vi "Log State JKI.vi"(0 "Current State In":string, 5 "Arguments In":string, 7 "Error In (no error)":errorcluster, 9 "StatesToIgnore":string[](array[string]), 11 "StatesForTraceLevel":string[](array[string]), 13 "EnableLogging?":bool) -> (6 "Current State":string, 8 "Arguments":string)   [LabVIEW 2020, in "TaskfileRunner Tool.lvlib"]
doc: "Log the state and arguments of the current state and also the error of the previous state of the JKI State Machine 2024 usually using the DEBUG log level.\nStates that are listed in the StatesForTraceLevel Input are logged with a log level of TRACE.\nStates that are listed in the StatesToIgnore are not logged.\n\nIt is important to use the JKI State Machine 2024"
uses:
  <vilib>/Utility/error.llb/DialogType.ctl
  16354a92-b9ac-49f3-ab46-e17f0121f75c.vi
  3b7a71ad-25d6-447f-a954-168ecec1f7c2.vi
  16354a92-b9ac-49f3-ab46-e17f0121f75c.vi/ff40df25-0e41-4205-825d-56c19dc320b6.vi
  3b7a71ad-25d6-447f-a954-168ecec1f7c2.vi/ff40df25-0e41-4205-825d-56c19dc320b6.vi
  <vilib>/Utility/Debug Log/Display.vi
  <vilib>/regexp/Match Regular Expression.xnode
  TaskfileRunner Tool.lvlib
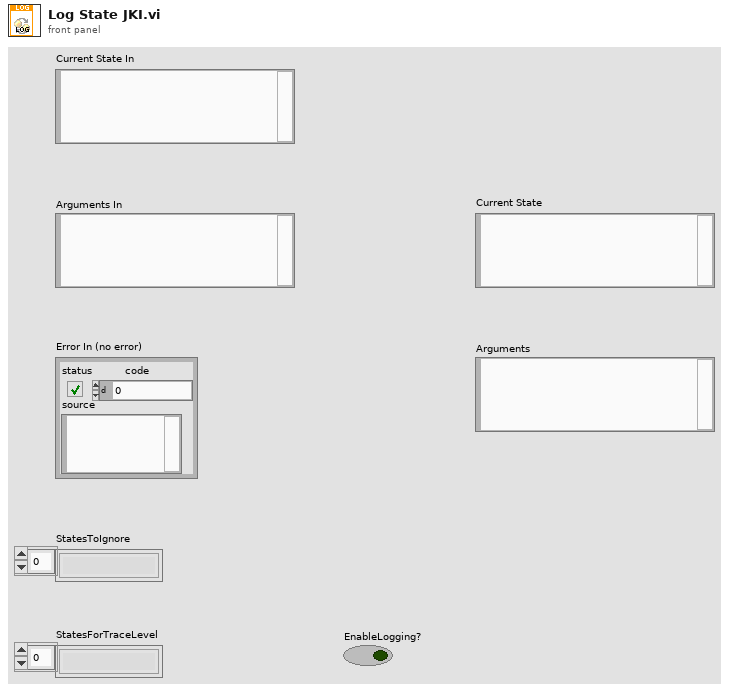
[diagram p1: front panel]
types:
  T1 = typedef "DialogType.ctl" = u16
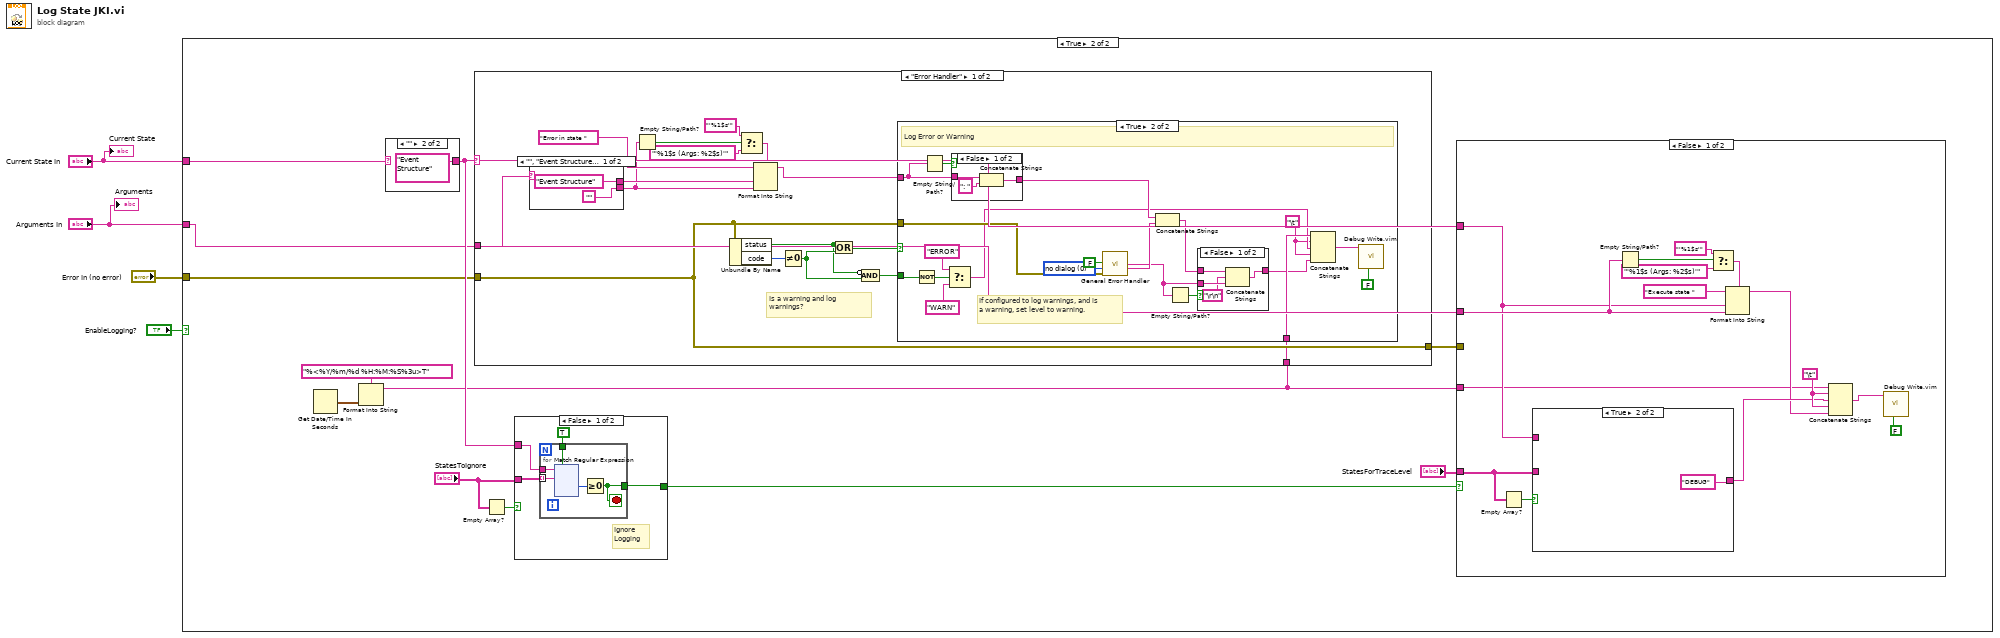
[diagram p0: block diagram]
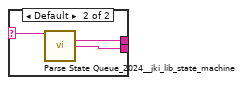
[diagram p6: hidden frame]
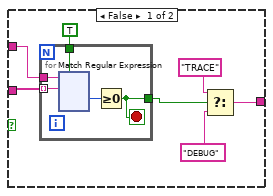
[diagram p10: hidden frame]
diagram:
  n1 = case shown="True" "EnableLogging?" {
    tunnel: "Current State In" -> [_ w12]
    tunnel: "Arguments In" -> [_ w11]
    tunnel: "Error In (no error)" -> [_ w10]
    frame False {
    }
    frame True {
      n2 = Get Date/Time In Seconds() -> (seconds since 1Jan1904=w7:timestamp)
      n3 = Format Into String(format string="%<%Y/%m/%d %H:%M:%S%3u>T", w7) -> (resulting string=w5:string)  [unwired: 2 in, 1 out]
      n4 = case shown="\"\"" w12 {
        selector: w12 -> [w68 _]
        tunnel: [w68 "Event Structure"] -> w14
        frame Default {
        }
        frame "" {
        }
      }
      n5 = case shown="\"Error Handler\"" w14 {
        tunnel: w11 -> [w30 _]
        tunnel: w10 -> [w18 w67]
        tunnel: [w18 w67] -> w8
        tunnel: w5 -> [w17 _]
        frame "Error Handler" {
          # "Is a warning and log warnings?"
          n6 = case shown="\"\", \"Event Structure\"" w30 {
            selector: w30 -> [_ w64]
            tunnel: ["Event Structure" ("Current State") w66] -> w32
            tunnel: ["" w65] -> w29
            frame "", "Event Structure" {
            }
            frame Default {
              n7 = call <vilib>:"Parse State Queue_2024__jki_lib_state_machine.vi"("State Queue"=w64) -> ("Current State"=w66:string, "Arguments"=w65:string)  [unwired: 12 in, 1 out]
            }
          }
          n8 = Empty String/Path?(string/path=w29) -> (empty?=w28:bool)
          n9 = Unbundle By Name(w18) -> ("status"=w22:bool, "code"=w24:i32)
          n10 = Select(t="'%1$s'" ("format string"), s=w28, f="'%1$s (Args: %2$s)'" ("format string")) -> (s? t:f=w25:string)
          n11 = Format Into String(format string=w25, initial string="Error in state ", w32, w29) -> (resulting string=w19:string)  [unwired: 1 in, 1 out]
          n12 = Not Equal To 0?(x=w24) -> (x != 0?=w23:bool)
          n13 = Or(x=w22, y=w23) -> (x .or. y?=w20:bool)
          n14 = Compound Arithmetic op=AND(invert w22, w23) -> (w21:bool)
          n15 = case shown="True" w20 {
            tunnel: w18 -> [_ w47]
            tunnel: w21 -> [_ w52]
            tunnel: w19 -> [_ w50]
            tunnel: w17 -> [_ w38]
            frame False {
              # "No error/not configured to log warnings, do nothing."
            }
            frame True {
              w36 = "\t"
              w46 = T1 0 items=["no dialog", "OK message", "continue or stop message", "OK message + warnings", "continue/stop + warnings"] ("type of dialog (OK msg:1)")
              # "If configured to log warnings, and is a warning, set level to warning."
              # "Log Error or Warning"
              n16 = Not(x=w52) -> (.not. x?=w51:bool)
              n17 = Empty String/Path?(string/path=w50) -> (empty?=w48:bool)
              n18 = Select(t="ERROR", s=w51, f="WARN") -> (s? t:f=w37:string)
              n19 = case shown="False" w48 {
                tunnel: w50 -> [w60 w61]
                tunnel: [w58 w61] -> w49
                frame False {
                  n20 = Concatenate Strings(w60, ": " ("string")) -> (w58:string)
                }
                frame True {
                }
              }
              n21 = call <vilib>:"General Error Handler.vi"("search ni.com link visible?(T)"=FALSE, "type of dialog (OK msg:1)"=w46, "error in (no error)"=w47) -> ("source out"=w42:string, "message"=w44:string)  [unwired: 8 in, 3 out]
              n22 = Concatenate Strings(w49, w44) -> (w34:string)
              n23 = Empty String/Path?(string/path=w42) -> (empty?=w43:bool)
              n24 = case shown="False" w43 {
                tunnel: w42 -> [w54 _]
                tunnel: [w56 w57] -> w35
                tunnel: w34 -> [w55 w57]
                frame False {
                  n25 = Concatenate Strings(w55, "\r\n", w54) -> (w56:string)
                }
                frame True {
                }
              }
              n26 = Concatenate Strings(w38, w36, w37, w36, w35) -> (w33:string)
              n27 = call "Debug Write.vim"("include timestamp? (F)"=FALSE, "value"=w33) -> ()  [unwired: 9 in, 1 out]
            }
          }
        }
        frame Default {
        }
      }
      n28 = Empty Array?(array="StatesToIgnore") -> (empty?=w16:bool)
      n29 = case shown="False" w16 {
        tunnel: "StatesToIgnore" -> [w73 _]
        tunnel: w14 -> [w72 _]
        tunnel: [w70 _] -> w13
        frame False {
          # "Ignore\nLogging"
          n30 = for {
            tunnel: [w77] -> w70
            tunnel: w73 -> [w76] mode=indexing
            tunnel: w72 -> [w75]
            tunnel: TRUE ("ignore case? (F)") -> [w74]
            stop <- w77 stop-if-true
            n31 = xnode "Match Regular Expression"("input string"=w75, "regular expression"=w76, "ignore case? (F)"=w74) -> ("offset past match"=w78:i32)  [unwired: 3 in, 4 out]
            n32 = Greater Or Equal To 0?(x=w78) -> (x >= 0?=w77:bool)
          }
        }
        frame True {
        }
      }
      n33 = case shown="False" w13 {
        tunnel: w14 -> [w200 _]
        tunnel: w11 -> [w201 _]
        tunnel: "StatesForTraceLevel" -> [w199 _]
        tunnel: w8 -> [_ _]
        tunnel: w5 -> [w193 _]
        frame False {
          w197 = "\t"
          n34 = Empty Array?(array=w199) -> (empty?=w207:bool)
          n35 = case shown="True" w207 {
            tunnel: w199 -> [w213 _]
            tunnel: w200 -> [w212 _]
            tunnel: [w214 "DEBUG"] -> w196
            frame False {
              n36 = for {
                tunnel: [w218] -> w211
                tunnel: w213 -> [w217] mode=indexing
                tunnel: w212 -> [w216]
                tunnel: TRUE ("ignore case? (F)") -> [w215]
                stop <- w218 stop-if-true
                n37 = xnode "Match Regular Expression"("input string"=w216, "regular expression"=w217, "ignore case? (F)"=w215) -> ("offset past match"=w219:i32)  [unwired: 3 in, 4 out]
                n38 = Greater Or Equal To 0?(x=w219) -> (x >= 0?=w218:bool)
              }
              n39 = Select(t="TRACE", s=w211, f="DEBUG") -> (s? t:f=w214:string)
            }
            frame True {
            }
          }
          n40 = Empty String/Path?(string/path=w201) -> (empty?=w203:bool)
          n41 = Select(t="'%1$s'" ("format string"), s=w203, f="'%1$s (Args: %2$s)'" ("format string")) -> (s? t:f=w206:string)
          n42 = Format Into String(format string=w206, initial string="Execute state ", w200, w201) -> (resulting string=w195:string)  [unwired: 1 in, 1 out]
          n43 = Concatenate Strings(w193, w197, w196, w197, w195) -> (w194:string)
          n44 = call "Debug Write.vim"("include timestamp? (F)"=FALSE, "value"=w194) -> ()  [unwired: 9 in, 1 out]
        }
        frame True {
        }
      }
    }
  }
  "Current State" <- "Current State In"
  "Arguments" <- "Arguments In"
